vi "graph_cursors_centerize.vi"(9 "centerize?":bool, 10 "x-axis array":dbl[](array[numeric]), 11 "XYGraph in":refnum<vi>) -> ()   [LabVIEW 2020]
panel:
  out "Array":T1(array[cluster])
  out "cursor x positions":dbl[](array[numeric])
  out "X Scale.Range:Minimum":dbl
  out "X Scale.Range:Maximum":dbl
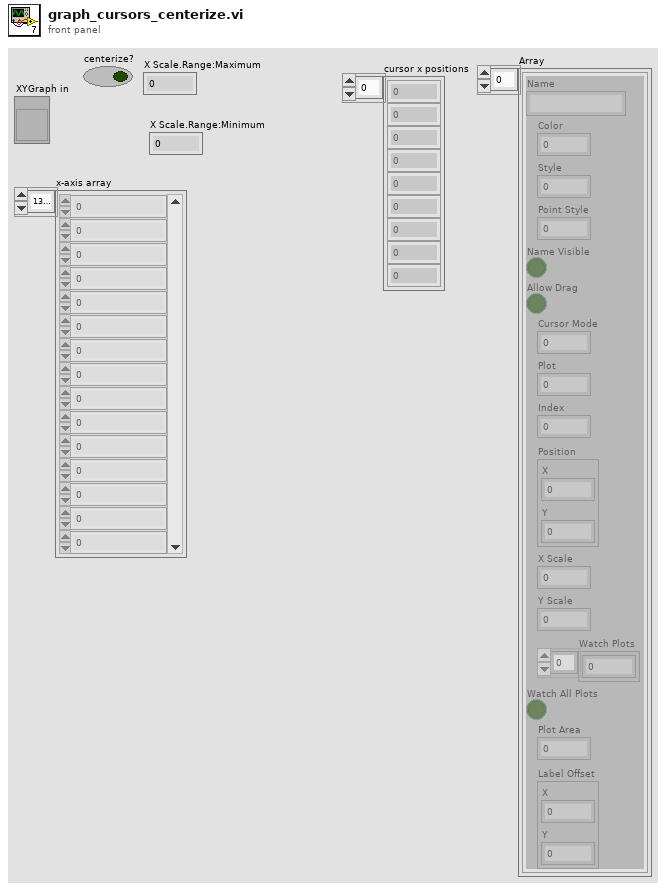
[diagram p1: front panel]
types:
  T1 = cluster{"Name":string, "Color":u32, "Style":u8, "Point Style":u8, "Name Visible":bool, "Allow Drag":bool, "Cursor Mode":u32, "Plot":i32, "Index":i32, "Position":cluster{"X":dbl, "Y":dbl}, "X Scale":u32, "Y Scale":u32, "Watch Plots":i32[], "Watch All Plots":bool, "Plot Area":i32, "Label Offset":cluster{"X":dbl, "Y":dbl}}[]
  T2 = typedef "LVCursorListTypeDef.ctl" = cluster{"Name":string, "Color":u32, "Style":u8, "Point Style":u8, "Name Visible":bool, "Allow Drag":bool, "Cursor Mode":u32, "Plot":i32, "Index":i32, "Position":cluster{"X":dbl, "Y":dbl}, "X Scale":u32, "Y Scale":u32, "Watch Plots":i32[], "Watch All Plots":bool, "Plot Area":i32, "Label Offset":cluster{"X":dbl, "Y":dbl}}[]
  T3 = cluster{"Name":string, "Color":u32, "Style":u8, "Point Style":u8, "Name Visible":bool, "Allow Drag":bool, "Cursor Mode":u32, "Plot":i32, "Index":i32, "Position":cluster{"X":dbl, "Y":dbl}, "X Scale":u32, "Y Scale":u32, "Watch Plots":i32[], "Watch All Plots":bool, "Plot Area":i32, "Label Offset":cluster{"X":dbl, "Y":dbl}}
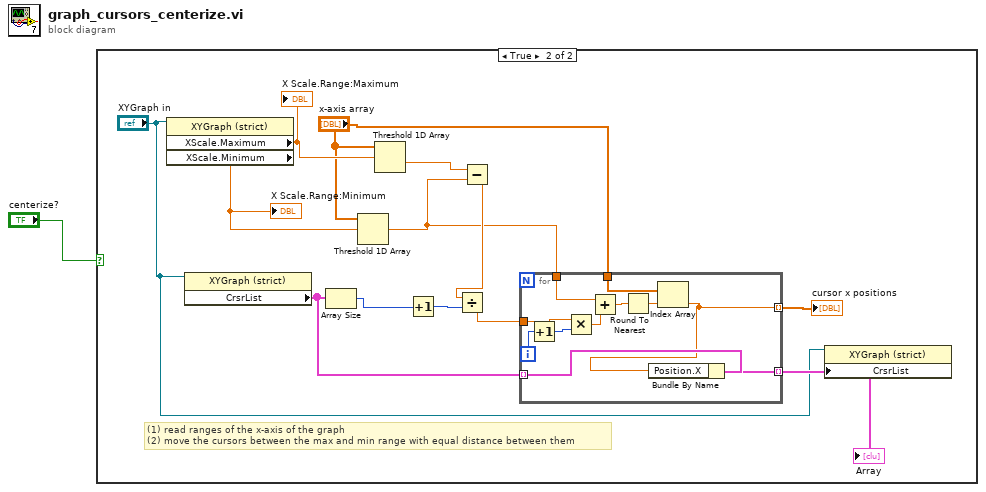
[diagram p0: block diagram]
diagram:
  n1 = case shown="True" "centerize?" {
    frame False {
    }
    frame True {
      # "(1) read ranges of the x-axis of the graph\n(2) move the cursors between the max and min range with equal distance between them"
      n2 = property on="Property Node" class="XYGraph (strict)"(reference="XYGraph in") -> ("XScale.Maximum"=w14:dbl, "XScale.Minimum"=w13:dbl)  [unwired: 1 in, 2 out]
      "X Scale.Range:Maximum" <- w14
      "X Scale.Range:Minimum" <- w13
      n3 = property class="XYGraph (strict)"(reference="XYGraph in") -> ("CrsrList"=w8:T2)  [unwired: 1 in, 2 out]
      n4 = Array Size(array=w8) -> (size(s)=w11:i32)
      n5 = Threshold 1D Array(2:w13, 3:"x-axis array") -> (0:w4:dbl)  [unwired: 1 in]
      n6 = Threshold 1D Array(2:w14, 3:"x-axis array") -> (0:w5:dbl)  [unwired: 1 in]
      n7 = Increment(x=w11) -> (x+1=w10:i32)
      n8 = Subtract(x=w5, y=w4) -> (x-y=w12:dbl)
      n9 = Divide(x=w12, y=w10) -> (x/y=w9:dbl)
      n10 = for {
        tunnel: w4 -> [w25]
        tunnel: w9 -> [w24]
        tunnel: w8 -> [w20] mode=indexing
        tunnel: [w19] -> w7 mode=indexing
        tunnel: [w15] -> w2 mode=indexing
        tunnel: "x-axis array" -> [w16]
        i -> [w23]
        n11 = Increment(x=w23) -> (x+1=w22:i32)
        n12 = Multiply(x=w24, y=w22) -> (x*y=w21:dbl)
        n13 = Add(x=w25, y=w21) -> (x+y=w18:dbl)
        n14 = Round To Nearest(number=w18) -> (nearest integer value=w17:dbl)
        n15 = Index Array(array=w16, index=w17) -> (element=w15:dbl)
        n16 = Bundle By Name(cluster=w20, "Position.X"=w15) -> (w19:T3)
      }
      "cursor x positions" <- w2
      "Array" <- w7
      n17 = property class="XYGraph (strict)"(reference="XYGraph in", "CrsrList"=w7) -> ()  [unwired: 1 in, 2 out]
    }
  }
